vi "atcs_getSample_LoopTimems.vi"(8 "error in (no error)":errorcluster, 11 "LoopTime_ms_Ctl":T1) -> (0 "error out":errorcluster, 2 "function return":i32, 3 "LoopTime_ms_Ctl out":T1)   [LabVIEW 2016, in "SALLV_atcs.lvlib"]
doc: "int atcs_shm_getSample_LoopTime_msLV(atcs_LoopTime_msLV *LoopTime_ms_Ctl );"
uses:
  SALLV_atcs.lvlib
  DataTypes/LoopTime_ms.ctl
  SALLV_atcs.so
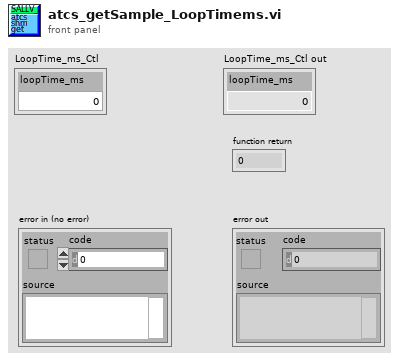
[diagram p1: front panel]
types:
  T1 = typedef "SALLV_atcs.lvlib/LoopTime_ms.ctl" = cluster{"loopTime_ms":dbl}
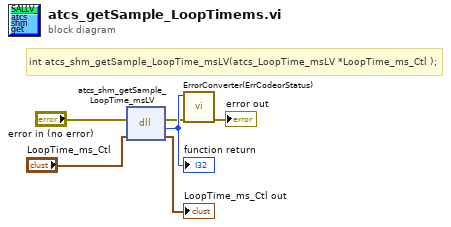
[diagram p0: block diagram]
diagram:
  # "int atcs_shm_getSample_LoopTime_msLV(atcs_LoopTime_msLV *LoopTime_ms_Ctl );"
  n1 = dll-call lib="home/andres/Desktop/SALLV_atcs/SALLV_atcs.*" fn="atcs_shm_getSample_LoopTime_msLV"(error in="error in (no error)", "LoopTime_ms_Ctl"="LoopTime_ms_Ctl") -> (error out=w2:errorcluster, w6:i32, "LoopTime_ms_Ctl"=→"LoopTime_ms_Ctl out":T1)  [unwired: 2 in, 1 out]
  "function return" <- w6
  n2 = call "ErrorConverter(ErrCodeorStatus).vi"("error in (no error)"=w2, "error code"=w6) -> ("error out"=→"error out":errorcluster)  [unwired: 9 in]
